vi "TSP_GA Solver.vi"(1 "pop_size":dbl=100.0, 2 "Number of Iterative":dbl) -> ()   [LabVIEW 2016]
panel:
  out "Numeric":i32
  out "error out":errorcluster
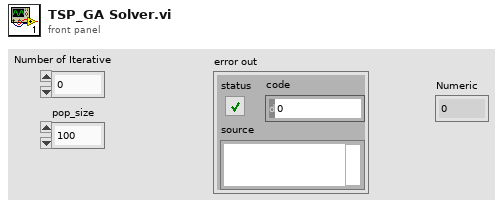
[diagram p1: front panel]
types:
  T1 = cluster{"Positions XY":dbl[][], "Optimal Path":dbl[], "Total Dist":dbl}
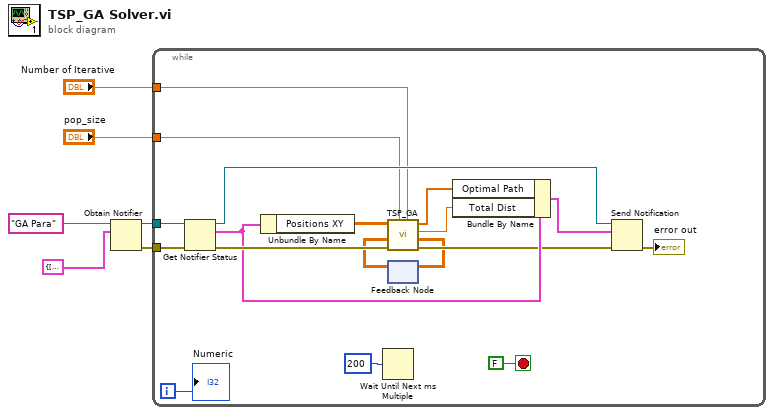
[diagram p0: block diagram]
diagram:
  n1 = Obtain Notifier(name (unnamed)="GA Para", notification data type=T1 {"Positions XY"=[], "Optimal Path"=[], "Total Dist"=0.0}) -> (notifier out=w5:refnum<notifier>, error out=w4:errorcluster)  [unwired: 2 in, 1 out]
  n2 = while {
    tunnel: w5 -> [w22]
    tunnel: w4 -> [w21]
    tunnel: "pop_size" -> [w9]
    tunnel: "Number of Iterative" -> [w8]
    i -> [w7]
    stop <- FALSE stop-if-true
    n3 = Get Notifier Status(notifier=w22, error in (no error)=w21) -> (notifier out=w13:refnum<notifier>, current notification=w18:T1, error out=w20:errorcluster)  [unwired: 2 out]
    n4 = Unbundle By Name(w18) -> ("Positions XY"=w19:dbl[][])
    n5 = Wait Until Next ms Multiple(millisecond multiple=u32 200 ("等待时间（毫秒）")) -> ()  [unwired: 1 out]
    n6 = feedback #1() -> (w10:dbl[][])  [unwired: 1 in]
    n7 = call "TSP_GA.vi"("Number of Iterative"=w8, "pop_size"=w9, "error in"=w20, "Pop in"=w10, "xy"=w19) -> ("error out"=w15:errorcluster, "pop out"=w11:dbl[][], "min dist"=w16:dbl, "opt_rte"=w17:dbl[])  [unwired: 2 in, 1 out]
    n8 = feedback-in #1(w11) -> ()
    n9 = Bundle By Name(cluster=w18, "Optimal Path"=w17, "Total Dist"=w16) -> (w12:T1)
    n10 = Send Notification(notification=w12, notifier=w13, error in (no error)=w15) -> (error out=→"error out":errorcluster)  [unwired: 1 out]
    "Numeric" <- w7
  }
